vi "Test Open Close.vi"(8 "error in (no error)":errorcluster, 11 "Instrument.Oxford1820 in":refnum<class "Instrument.Oxford1820.lvclass">) -> (0 "error out":errorcluster, 3 "Instrument.Oxford1820 out":refnum<class "Instrument.Oxford1820.lvclass">)   [LabVIEW 2016, in "Instrument.Oxford1820.lvclass"]
uses:
  Instrument.Oxford1820.lvclass
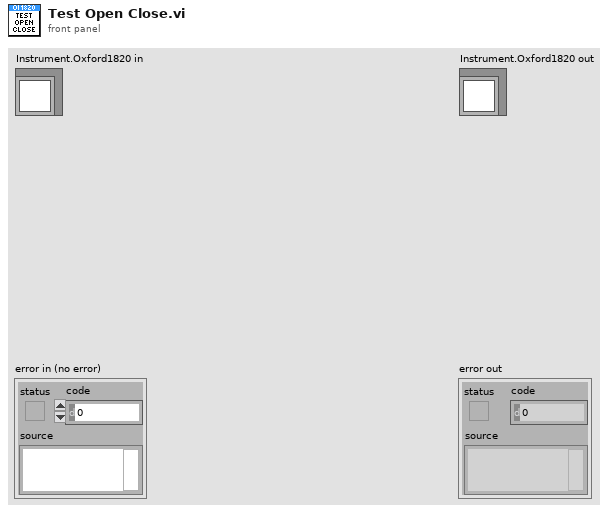
[diagram p1: front panel]
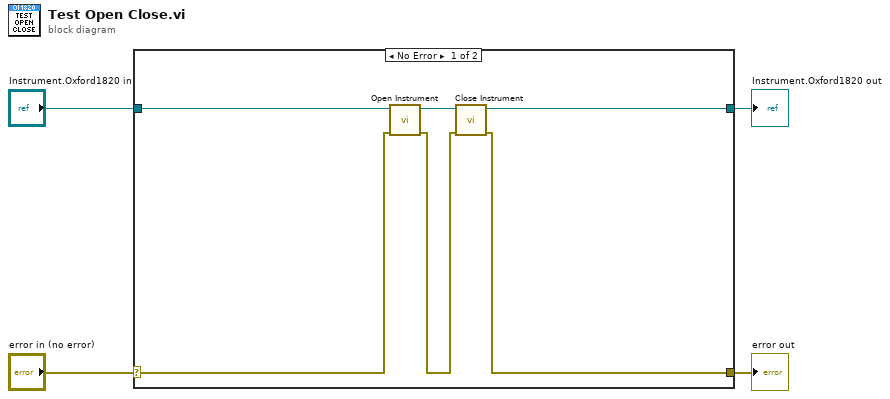
[diagram p0: block diagram]
diagram:
  n1 = case shown="No Error" "error in (no error)" {
    selector: "error in (no error)" -> [w7 w12]
    tunnel: [w5 w12] -> w3
    tunnel: [w8 w11] -> w1
    tunnel: "Instrument.Oxford1820 in" -> [w9 w11]
    frame No Error {
      n2 = call-dynamic "Open Instrument.vi"("error in (no error)"=w7, "Instrument.Oxford1820 in"=w9) -> ("error out"=w6:errorcluster, "Instrument.Oxford1820 out"=w10:refnum<class "Instrument.Oxford1820.lvclass">)  [unwired: 8 in]
      n3 = call-dynamic "Close Instrument.vi"("error in (no error)"=w6, "Instrument.Oxford1820 in"=w10) -> ("error out"=w5:errorcluster, "Instrument.Oxford1820 out"=w8:refnum<class "Instrument.Oxford1820.lvclass">)  [unwired: 8 in]
    }
    frame Error {
    }
  }
  "error out" <- w3
  "Instrument.Oxford1820 out" <- w1
